vi "ASK_2_receiver.vi"() -> ()   [LabVIEW 2015]
panel:
  in  "x":i16
  out "De":dbl[](graph)
  in  "Numeric":i32
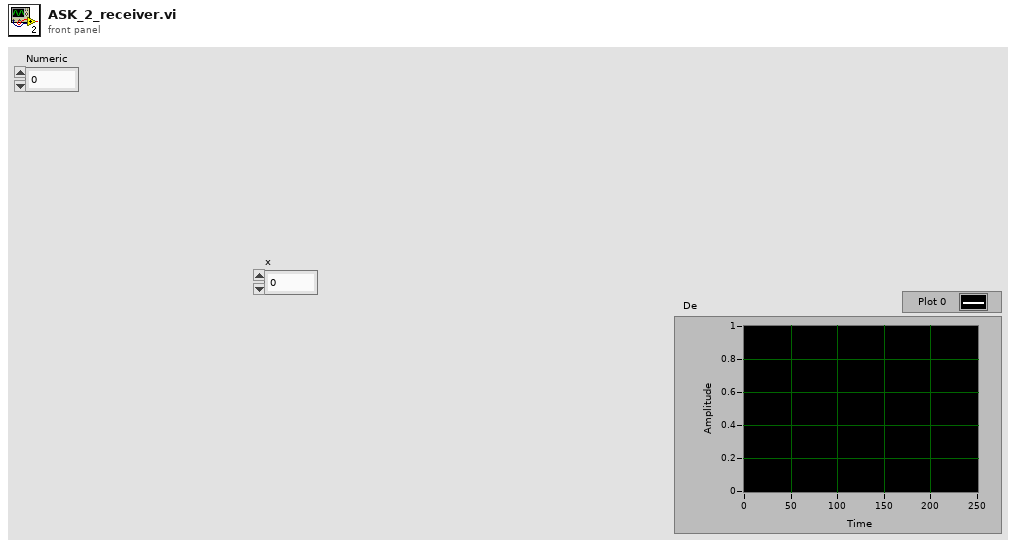
[diagram p1: front panel]
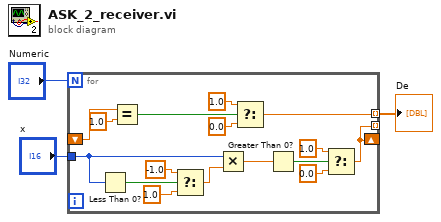
[diagram p0: block diagram]
diagram:
  n1 = for {
    N: "Numeric" -> [_]
    tunnel: [w11] -> _ mode=indexing
    shift-right: [w11] -> _
    shift-left: _ -> [w10]
    tunnel: [w5] -> w2 mode=indexing
    tunnel: "x" -> [w4]
    n2 = Less Than 0?(x=w4) -> (x < 0?=w19:bool)
    n3 = Equal?(x=w10, y=1.0) -> (x = y?=w8:bool)
    n4 = Select(t=-1.0, s=w19, f=1.0) -> (s? t:f=w16:dbl)
    n5 = Multiply(x=w4, y=w16) -> (x*y=w15:dbl)
    n6 = Select(t=1.0, s=w8, f=0.0) -> (s? t:f=w5:dbl)
    n7 = Greater Than 0?(x=w15) -> (x > 0?=w14:bool)
    n8 = Select(t=1.0, s=w14, f=0.0) -> (s? t:f=w11:dbl)
  }
  "De" <- w2
